vi "Write ini.vi"(8 "error in (no error)":errorcluster, 11 "Sett data":T1={"Filter"=0, "Gain"=0.0, "Bit rate"=0.0, "ISO/IEC w "=enum."14443 Type A", "BI"={"R"=0.0, "C"=0.0, "L"=0.0}, "BM"={"R"=0.0, "C"=0.0, "L"=0.0}, "M"={"Метка"=4, "Считыветель"=4}, "Type noise"=enum."Гауссовский шум", "Link"=enum."UPLINK", "Noise attenuator"=0.0, "Signal gain"=1.0, "Distance"=0.0} {"Distance" scale=0.0..10.0; "Signal gain" min=1.0 max=100.0 step=1.0 scale=1.0..30.0; "Noise attenuator" scale=0.01..1.01; "M"."Считыветель" min=4 max=128 step=4; "M"."Метка" min=4 max=128 step=4; "Bit rate" min=4.0 max=128.0 step=4.0}) -> (0 "error out":errorcluster)   [LabVIEW 2019]
uses:
  TypeDef/Sett data.ctl
  TypeDef/ISO.ctl
  TypeDef/Noise.ctl
  TypeDef/Link.ctl
  <vilib>/Utility/config.llb/Write Key (I32).vi
  <vilib>/Utility/config.llb/Write Key (Double).vi
  <vilib>/Utility/config.llb/NI_LVConfig.lvlib
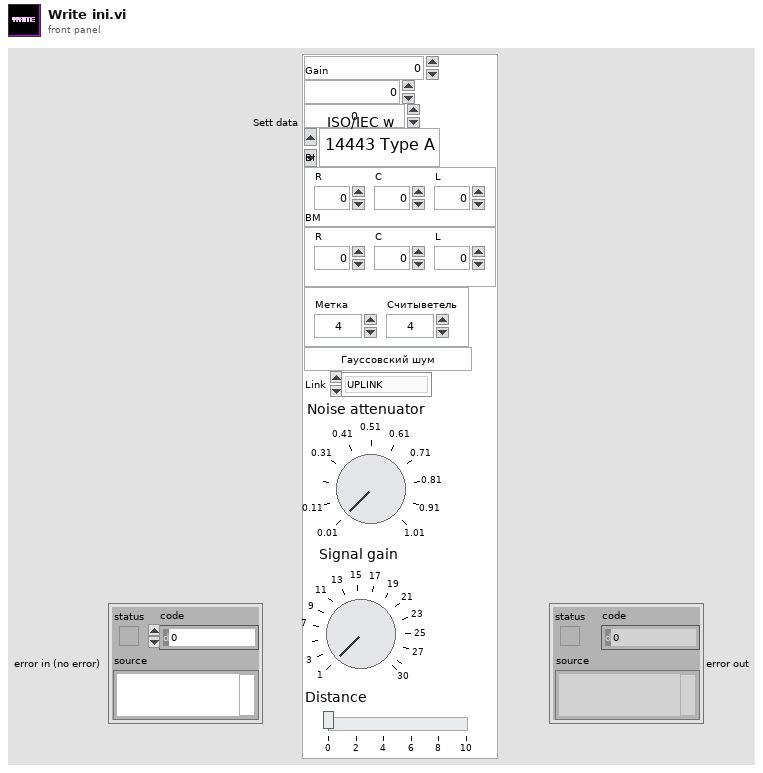
[diagram p1: front panel]
types:
  T1 = typedef "Sett data.ctl" = cluster{"Filter":i32, "Gain":dbl, "Bit rate":dbl, "ISO/IEC w ":T2, "BI":cluster{"R":dbl, "C":dbl, "L":dbl}, "BM":cluster{"R":dbl, "C":dbl, "L":dbl}, "M":cluster{"Метка":i64, "Считыветель":i64}, "Type noise":T3, "Link":T4, "Noise attenuator":dbl, "Signal gain":dbl, "Distance":dbl}
  T2 = typedef "ISO.ctl" = enum16{"14443 Type A", "14443 Type B", "Felica", "15693"}
  T3 = typedef "Noise.ctl" = enum16{"Гауссовский шум", "Белый шум"}
  T4 = typedef "Link.ctl" = enum16{"UPLINK", "DOWNLINK"}
  T5 = typedef "NI_LVConfig.lvlib/Config Data RefNum.ctl" = refnum<k1>
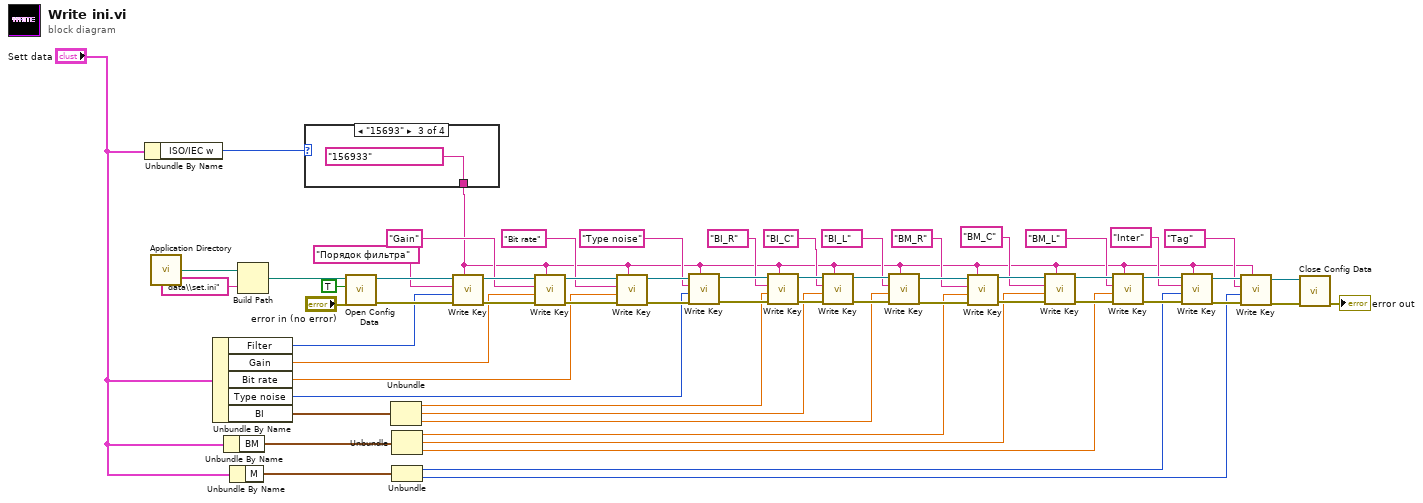
[diagram p0: block diagram]
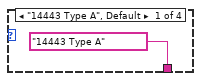
[diagram p2: hidden frame]
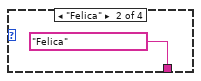
[diagram p3: hidden frame]
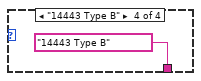
[diagram p4: hidden frame]
diagram:
  n1 = Unbundle By Name("Sett data") -> ("ISO/IEC w"=w55:T2)
  n2 = call <vilib>:"Application Directory.vi"() -> ("Application Directory"=w62:path)
  n3 = Unbundle By Name("Sett data") -> ("Filter"=w44:i32, "Gain"=w41:dbl, "Bit rate"=w40:dbl, "Type noise"=w38:T3, "BI"=w37:cluster{"R":dbl, "C":dbl, "L":dbl})
  n4 = Unbundle By Name("Sett data") -> ("BM"=w14:cluster{"R":dbl, "C":dbl, "L":dbl})
  n5 = Unbundle By Name("Sett data") -> ("M"=w12:cluster{"Метка":i64, "Считыветель":i64})
  n6 = Build Path(base path=w62, name or relative path="data\\set.ini") -> (appended path=w60:path)
  n7 = case shown="\"15693\"" w55 {
    tunnel: ["14443 Type A" "Felica" "156933" "14443 Type B"] -> w1
    frame "14443 Type A", Default {
    }
    frame "Felica" {
    }
    frame "15693" {
    }
    frame "14443 Type B" {
    }
  }
  n8 = call <vilib>:"Open Config Data.vi"("error in (no error)"="error in (no error)", "create file if necessary (T)"=TRUE, "configuration file path"=w60) -> ("error out"=w58:errorcluster, "refnum"=w54:T5)  [unwired: 6 in, 1 out]
  n9 = Unbundle(w37) -> ("R"=w17:dbl, "C"=w16:dbl, "L"=w15:dbl)
  n10 = Unbundle(w14) -> ("R"=w8:dbl, "C"=w7:dbl, "L"=w6:dbl)
  n11 = Unbundle(w12) -> ("Метка"=w5:i64, "Считыветель"=w4:i64)
  n12 = call-poly <vilib>:"Write Key.vi"("section"=w1, "error in (no error)"=w58, "value"=w44, "key"="Порядок фильтра", "refnum"=w54) -> ("error out"=w57:errorcluster, "refnum out"=w53:T5)  [unwired: 4 in, 1 out]
  n13 = call-poly <vilib>:"Write Key.vi"("section"=w1, "error in (no error)"=w57, "value"=w41, "key"="Gain", "refnum"=w53) -> ("error out"=w56:errorcluster, "refnum out"=w52:T5)  [unwired: 4 in, 1 out]
  n14 = call-poly <vilib>:"Write Key.vi"("section"=w1, "error in (no error)"=w56, "value"=w40, "key"="Bit rate", "refnum"=w52) -> ("error out"=w51:errorcluster, "refnum out"=w48:T5)  [unwired: 4 in, 1 out]
  n15 = call-poly <vilib>:"Write Key.vi"("section"=w1, "error in (no error)"=w51, "value"=w38, "key"="Type noise", "refnum"=w48) -> ("error out"=w50:errorcluster, "refnum out"=w49:T5)  [unwired: 4 in, 1 out]
  n16 = call-poly <vilib>:"Write Key.vi"("section"=w1, "error in (no error)"=w50, "value"=w17, "key"="BI_R", "refnum"=w49) -> ("error out"=w23:errorcluster, "refnum out"=w24:T5)  [unwired: 4 in, 1 out]
  n17 = call-poly <vilib>:"Write Key.vi"("section"=w1, "error in (no error)"=w23, "value"=w16, "key"="BI_C", "refnum"=w24) -> ("error out"=w35:errorcluster, "refnum out"=w36:T5)  [unwired: 4 in, 1 out]
  n18 = call-poly <vilib>:"Write Key.vi"("section"=w1, "error in (no error)"=w35, "value"=w15, "key"="BI_L", "refnum"=w36) -> ("error out"=w33:errorcluster, "refnum out"=w34:T5)  [unwired: 4 in, 1 out]
  n19 = call-poly <vilib>:"Write Key.vi"("section"=w1, "error in (no error)"=w33, "value"=w8, "key"="BM_R", "refnum"=w34) -> ("error out"=w31:errorcluster, "refnum out"=w32:T5)  [unwired: 4 in, 1 out]
  n20 = call-poly <vilib>:"Write Key.vi"("section"=w1, "error in (no error)"=w31, "value"=w7, "key"="BM_C", "refnum"=w32) -> ("error out"=w29:errorcluster, "refnum out"=w30:T5)  [unwired: 4 in, 1 out]
  n21 = call-poly <vilib>:"Write Key.vi"("section"=w1, "error in (no error)"=w29, "value"=w6, "key"="BM_L", "refnum"=w30) -> ("error out"=w27:errorcluster, "refnum out"=w28:T5)  [unwired: 4 in, 1 out]
  n22 = call-poly <vilib>:"Write Key.vi"("section"=w1, "error in (no error)"=w27, "value"=w5, "key"="Inter", "refnum"=w28) -> ("error out"=w25:errorcluster, "refnum out"=w26:T5)  [unwired: 4 in, 1 out]
  n23 = call-poly <vilib>:"Write Key.vi"("section"=w1, "error in (no error)"=w25, "value"=w4, "key"="Tag", "refnum"=w26) -> ("error out"=w21:errorcluster, "refnum out"=w22:T5)  [unwired: 4 in, 1 out]
  n24 = call <vilib>:"Close Config Data.vi"("error in (no error)"=w21, "refnum"=w22) -> ("error out"=→"error out":errorcluster)  [unwired: 8 in, 1 out]
